vi "HandleFIFOsetting_5761.vi"(8 "timed out":bool, 11 "Value":u64) -> ()   [LabVIEW 2025]
uses:
  <vilib>/rvi/Emulation/niFpgaEmulationIsFPGAContextNoSignature.vi
  <vilib>/rvi/DataTransferAndStorage/Container/Common/niFpgaContainerGetUniqueNameForEmu.vi
  <vilib>/rvi/Memory/Memory_Emulation/niFpgaMemoryEmulationCacheClearOnFirstRun.vi
  <vilib>/rvi/Memory/Memory_Emulation/nirvimemoryEmulationManagerCache_MakeExclusive.vi
  <vilib>/rvi/Memory/Memory_Emulation/niFpgaMemoryEmulationValidateCache.vi
  <vilib>/rvi/Memory/Memory_Emulation/nirvimemoryEmulationManagerCache_InsertValue.vi
  <vilib>/Utility/error.llb/Clear Errors.vi
  <vilib>/rvi/Memory/Memory_Emulation/nirvimemoryEmulationManagerCache_ReleaseExclusive.vi
  <vilib>/rvi/Memory/Memory_Emulation/nirvimemoryEmulationManagerCache_GetValue.vi
  <vilib>/rvi/Memory/Memory_Emulation/nirvimemoryEmulationManagerCache_SetValue.vi
  <vilib>/rvi/Emulation/niFpgaProcessEmulError.vi
  <vilib>/rvi/Emulation/niFpgaSctlEmulationGetInTimedLoop.vi
  <vilib>/rvi/DataTransferAndStorage/Container/XNode/niFpgaContainer.xnode
  <vilib>/rvi/DataTransferAndStorage/Register/Emulation/niFpgaRegisterEmulation.vi
  <vilib>/rvi/FXPMathLib/FxpInterpret/XNode/nifxpmath_Interpret.xnode
  fpga_settings.ctl
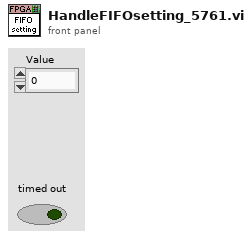
[diagram p1: front panel]
types:
  T1 = typedef "fpga_settings.ctl" = enum16{"Feedback Enable", "New FIR coeffs", "FIR shift", "Enable filter", "Set Downsample", "Downsample", "CIC Gain", "Record length", "Trigger samples", "Quiet time", "a_am", "b_am", "Use fixed delay", "fixed sin_fi", "fixed cos_fi", "Ki*Tau", "Kp", "Kd_Tau", "Fi_start", "Fi_delta", "DC_offs 0", "DC_offs 1", "DC_offs 2", "DC_offs 3", "Ki*Tau am", "Kp am", "Kd_Tau am", "Feedback AM", "Trigger delay", "Feedback delay", "Setpoint enable", "Beam enable", "Samples to acquire", "Cavity Enable", "Cavity C1", "Cavity C2", "Cavity C3", "Cavity C4", "Cavity C5", "Input delay", "Ki*Tau Q", "Kp Q", "Kd_Tau Q", "Adaptive FF enable", "Feedforward a0", "Feedforward b0", "FF src adress", "FF dest adress", "Output scale", "Input scale", "Host scale", "FF_IIR b0", "FF_IIR b1", "FF_IIR b2", "FF_IIR-a1", "FF_IIR-a2", "Enable HW trigger", "Virtual cavity", "Samples to skip", "Samples to skip 2", "Samples to skip 3", "Cavity C3_2", "Cavity C4_2", "Cavity C5_2", "Cavity C3_3", "Cavity C4_3", "Cavity C5_3", "Cavity_w0_dt", "Piezo setting", "Quench t0", "Quench tau set", "Quench enabled", "Quench reset", "PID enabled I", "PID enabled Q", "Cavity filter a", "Cavity filter b", "Disable e(n)", "FF e(n) src address", "FF first address", "FF last address", "FF PID first address", "FF PID last address", "Amp IIR b0", "Amp IIR b1", "Amp IIR b2", "Amp IIR-a1", "Amp IIR-a2", "Adaptation factor", "Inv Amp LP b0", "Inv Amp LP b1", "Inv Amp LP b2", "Inv Amp LP-a1", "Inv Amp LP-a2", "Inv Amp c0", "Inv Amp c1", "Inv Amp c2", "Inv Amp c3", "Inv Amp c4", "Inv Amp -d1", "Inv Amp -d2", "Inv Amp -d3", "Inv Amp -d4", "w12_a", "w12_b", "w12_dt", "w12_scale", "dw_scale", "Extra output select", "Extra fi sin", "Extra fi cos", "Extra output scale", "Quench max output"}
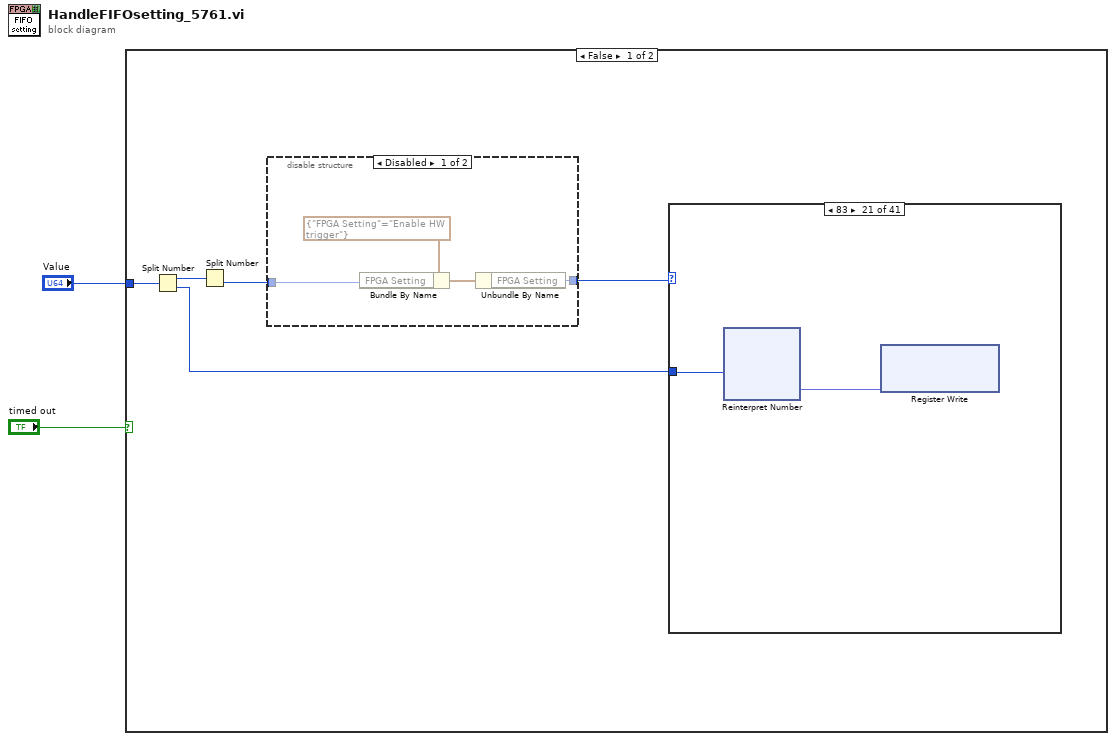
[diagram p0: block diagram]
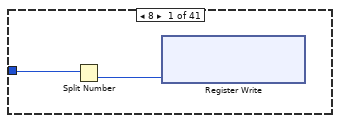
[diagram p3: hidden frame]
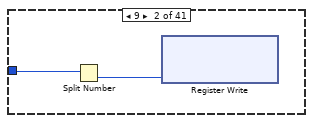
[diagram p4: hidden frame]
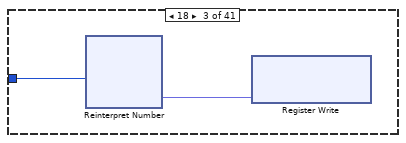
[diagram p5: hidden frame]
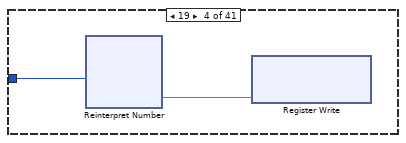
[diagram p6: hidden frame]
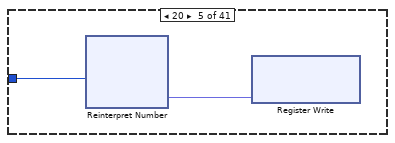
[diagram p7: hidden frame]
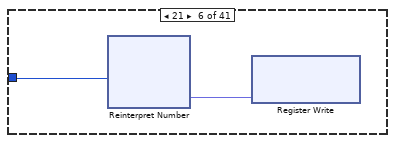
[diagram p8: hidden frame]
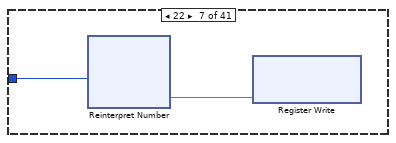
[diagram p9: hidden frame]
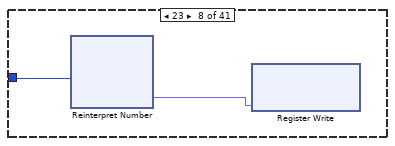
[diagram p10: hidden frame]
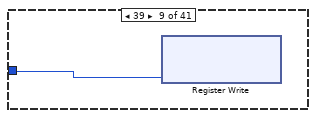
[diagram p11: hidden frame]
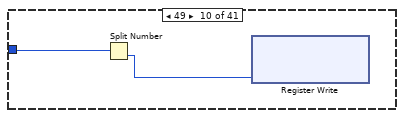
[diagram p12: hidden frame]
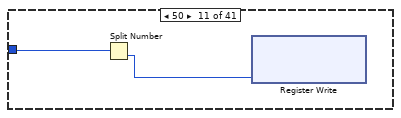
[diagram p13: hidden frame]
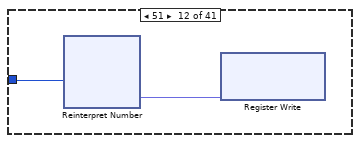
[diagram p14: hidden frame]
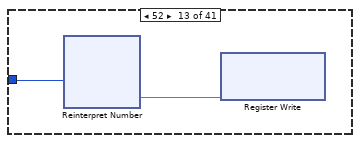
[diagram p15: hidden frame]
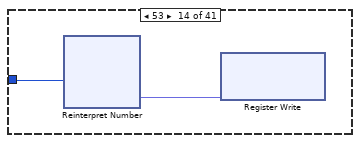
[diagram p16: hidden frame]
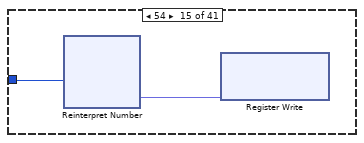
[diagram p17: hidden frame]
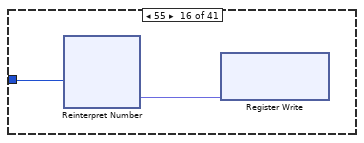
[diagram p18: hidden frame]
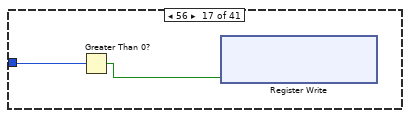
[diagram p19: hidden frame]
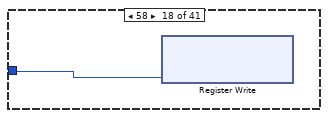
[diagram p20: hidden frame]
diagram:
  n1 = case shown="False" "timed out" {
    tunnel: "Value" -> [w7 _]
    frame False {
      n2 = Split Number(x=w7) -> (hi(x)=w6:u32, lo(x)=w3:u32)
      n3 = Split Number(x=w6) -> (lo(x)=w5:u16)  [unwired: 1 out]
      n4 = disable-structure shown="Disabled" {
        disable-tunnel: [w9 w12] -> w4
        disable-tunnel: w5 -> [w8 w12]
        frame Disabled {
          n5 = Bundle By Name(cluster=cluster{"FPGA Setting":T1} {"FPGA Setting"=enum."Enable HW trigger"}, "FPGA Setting"=w8) -> (w10:cluster{"FPGA Setting":T1})
          n6 = Unbundle By Name(w10) -> ("FPGA Setting"=w9:T1)
        }
        frame Enabled {
        }
      }
      n7 = case shown="83" w4 {
        tunnel: w3 -> [w14 w16 w18 w20 w22 w24 w26 w28 w29 w31 w33 w35 w37 w39 w41 w43 w45 w46 w47 w48 w50 w52 w54 w56 w58 w60 w62 w64 w66 w68 w70 w72 w74 w76 w78 w80 w82 w84 w86 w88 _]
        frame 8 {
          n8 = Split Number(x=w14) -> (lo(x)=w13:u16)  [unwired: 1 out]
          n9 = xnode ("Register Write")("Data"=w13) -> ()  [unwired: 1 in, 1 out]
        }
        frame 9 {
          n10 = Split Number(x=w16) -> (lo(x)=w15:u16)  [unwired: 1 out]
          n11 = xnode ("Register Write")("Data"=w15) -> ()  [unwired: 1 in, 1 out]
        }
        frame 18 {
          n12 = xnode "Reinterpret Number"("x"=w18) -> ("y"=w17:fxp<+/-,32,4>)
          n13 = xnode ("Register Write")("Data"=w17) -> ()  [unwired: 1 in, 1 out]
        }
        frame 19 {
          n14 = xnode "Reinterpret Number"("x"=w20) -> ("y"=w19:fxp<+/-,32,4>)
          n15 = xnode ("Register Write")("Data"=w19) -> ()  [unwired: 1 in, 1 out]
        }
        frame 20 {
          n16 = xnode "Reinterpret Number"("x"=w22) -> ("y"=w21:fxp<+/-,32,14>)
          n17 = xnode ("Register Write")("Data"=w21) -> ()  [unwired: 1 in, 1 out]
        }
        frame 21 {
          n18 = xnode "Reinterpret Number"("x"=w24) -> ("y"=w23:fxp<+/-,32,14>)
          n19 = xnode ("Register Write")("Data"=w23) -> ()  [unwired: 1 in, 1 out]
        }
        frame 22 {
          n20 = xnode "Reinterpret Number"("x"=w26) -> ("y"=w25:fxp<+/-,32,14>)
          n21 = xnode ("Register Write")("Data"=w25) -> ()  [unwired: 1 in, 1 out]
        }
        frame 23 {
          n22 = xnode "Reinterpret Number"("x"=w28) -> ("y"=w27:fxp<+/-,32,14>)
          n23 = xnode ("Register Write")("Data"=w27) -> ()  [unwired: 1 in, 1 out]
        }
        frame 39 {
          n24 = xnode ("Register Write")("Data"=w29) -> ()  [unwired: 1 in, 1 out]
        }
        frame 49 {
          n25 = Split Number(x=w31) -> (lo(x)=w30:u16)  [unwired: 1 out]
          n26 = xnode ("Register Write")("Data"=w30) -> ()  [unwired: 1 in, 1 out]
        }
        frame 50 {
          n27 = Split Number(x=w33) -> (lo(x)=w32:u16)  [unwired: 1 out]
          n28 = xnode ("Register Write")("Data"=w32) -> ()  [unwired: 1 in, 1 out]
        }
        frame 51 {
          n29 = xnode "Reinterpret Number"("x"=w35) -> ("y"=w34:fxp<+/-,32,2>)
          n30 = xnode "Register Write"("Data"=w34) -> ()  [unwired: 1 in, 1 out]
        }
        frame 52 {
          n31 = xnode "Reinterpret Number"("x"=w37) -> ("y"=w36:fxp<+/-,32,2>)
          n32 = xnode "Register Write"("Data"=w36) -> ()  [unwired: 1 in, 1 out]
        }
        frame 53 {
          n33 = xnode "Reinterpret Number"("x"=w39) -> ("y"=w38:fxp<+/-,32,2>)
          n34 = xnode "Register Write"("Data"=w38) -> ()  [unwired: 1 in, 1 out]
        }
        frame 54 {
          n35 = xnode "Reinterpret Number"("x"=w41) -> ("y"=w40:fxp<+/-,32,2>)
          n36 = xnode "Register Write"("Data"=w40) -> ()  [unwired: 1 in, 1 out]
        }
        frame 55 {
          n37 = xnode "Reinterpret Number"("x"=w43) -> ("y"=w42:fxp<+/-,32,2>)
          n38 = xnode "Register Write"("Data"=w42) -> ()  [unwired: 1 in, 1 out]
        }
        frame 56 {
          n39 = Greater Than 0?(x=w45) -> (x > 0?=w44:bool)
          n40 = xnode "Register Write"("Data"=w44) -> ()  [unwired: 1 in, 1 out]
        }
        frame 58 {
          n41 = xnode ("Register Write")("Data"=w46) -> ()  [unwired: 1 in, 1 out]
        }
        frame 59 {
          n42 = xnode ("Register Write")("Data"=w47) -> ()  [unwired: 1 in, 1 out]
        }
        frame 60 {
          n43 = xnode ("Register Write")("Data"=w48) -> ()  [unwired: 1 in, 1 out]
        }
        frame 83 {
          n44 = xnode "Reinterpret Number"("x"=w50) -> ("y"=w49:fxp<+/-,32,2>)
          n45 = xnode "Register Write"("Data"=w49) -> ()  [unwired: 1 in, 1 out]
        }
        frame 84 {
          n46 = xnode "Reinterpret Number"("x"=w52) -> ("y"=w51:fxp<+/-,32,2>)
          n47 = xnode "Register Write"("Data"=w51) -> ()  [unwired: 1 in, 1 out]
        }
        frame 85 {
          n48 = xnode "Reinterpret Number"("x"=w54) -> ("y"=w53:fxp<+/-,32,2>)
          n49 = xnode "Register Write"("Data"=w53) -> ()  [unwired: 1 in, 1 out]
        }
        frame 86 {
          n50 = xnode "Reinterpret Number"("x"=w56) -> ("y"=w55:fxp<+/-,32,2>)
          n51 = xnode "Register Write"("Data"=w55) -> ()  [unwired: 1 in, 1 out]
        }
        frame 87 {
          n52 = xnode "Reinterpret Number"("x"=w58) -> ("y"=w57:fxp<+/-,32,2>)
          n53 = xnode "Register Write"("Data"=w57) -> ()  [unwired: 1 in, 1 out]
        }
        frame 89 {
          n54 = xnode "Reinterpret Number"("x"=w60) -> ("y"=w59:fxp<+/-,32,2>)
          n55 = xnode "Register Write"("Data"=w59) -> ()  [unwired: 1 in, 1 out]
        }
        frame 90 {
          n56 = xnode "Reinterpret Number"("x"=w62) -> ("y"=w61:fxp<+/-,32,2>)
          n57 = xnode "Register Write"("Data"=w61) -> ()  [unwired: 1 in, 1 out]
        }
        frame 91 {
          n58 = xnode "Reinterpret Number"("x"=w64) -> ("y"=w63:fxp<+/-,32,2>)
          n59 = xnode "Register Write"("Data"=w63) -> ()  [unwired: 1 in, 1 out]
        }
        frame 92 {
          n60 = xnode "Reinterpret Number"("x"=w66) -> ("y"=w65:fxp<+/-,32,2>)
          n61 = xnode "Register Write"("Data"=w65) -> ()  [unwired: 1 in, 1 out]
        }
        frame 93 {
          n62 = xnode "Reinterpret Number"("x"=w68) -> ("y"=w67:fxp<+/-,32,2>)
          n63 = xnode "Register Write"("Data"=w67) -> ()  [unwired: 1 in, 1 out]
        }
        frame 94 {
          n64 = xnode "Reinterpret Number"("x"=w70) -> ("y"=w69:fxp<+/-,32,2>)
          n65 = xnode "Register Write"("Data"=w69) -> ()  [unwired: 1 in, 1 out]
        }
        frame 95 {
          n66 = xnode "Reinterpret Number"("x"=w72) -> ("y"=w71:fxp<+/-,32,2>)
          n67 = xnode "Register Write"("Data"=w71) -> ()  [unwired: 1 in, 1 out]
        }
        frame 96 {
          n68 = xnode "Reinterpret Number"("x"=w74) -> ("y"=w73:fxp<+/-,32,2>)
          n69 = xnode "Register Write"("Data"=w73) -> ()  [unwired: 1 in, 1 out]
        }
        frame 99 {
          n70 = xnode "Reinterpret Number"("x"=w76) -> ("y"=w75:fxp<+/-,32,2>)
          n71 = xnode "Register Write"("Data"=w75) -> ()  [unwired: 1 in, 1 out]
        }
        frame 100 {
          n72 = xnode "Reinterpret Number"("x"=w78) -> ("y"=w77:fxp<+/-,32,2>)
          n73 = xnode "Register Write"("Data"=w77) -> ()  [unwired: 1 in, 1 out]
        }
        frame 103 {
          n74 = xnode "Reinterpret Number"("x"=w80) -> ("y"=w79:fxp<+/-,32,12>)
          n75 = xnode ("Register Write")("Data"=w79) -> ()  [unwired: 1 in, 1 out]
        }
        frame 104 {
          n76 = xnode "Reinterpret Number"("x"=w82) -> ("y"=w81:fxp<+/-,32,14>)
          n77 = xnode ("Register Write")("Data"=w81) -> ()  [unwired: 1 in, 1 out]
        }
        frame 105 {
          n78 = xnode "Reinterpret Number"("x"=w84) -> ("y"=w83:fxp<+/-,32,26>)
          n79 = xnode "Register Write"("Data"=w83) -> ()  [unwired: 1 in, 1 out]
        }
        frame 106 {
          n80 = Split Number(x=w86) -> (lo(x)=w85:u16)  [unwired: 1 out]
          n81 = xnode "Register Write"("Data"=w85) -> ()  [unwired: 1 in, 1 out]
        }
        frame 107 {
          n82 = Split Number(x=w88) -> (lo(x)=w87:u16)  [unwired: 1 out]
          n83 = xnode "Register Write"("Data"=w87) -> ()  [unwired: 1 in, 1 out]
        }
        frame Default {
        }
      }
    }
    frame True {
    }
  }
